vi "Convert_ERDs_Brass.vi"(0 "New Header?":bool, 7 "Array":T7[](array[typedef]) {"ERD Number" format="%.0x"}, 11 "Error In":errorcluster) -> (4 "All_ERD_Data_Bundled_Brass":T1, 15 "Error Out":errorcluster)   [LabVIEW 2016]
doc: "This VI parses the data from ERDs in correct format, units, etc. It handles all hex to dec conversions, hex to enum, and hex to boolean conversions.\n\nIf Raw Data from ERD is blank string, then it will output values from shift register."
uses:
  Common/LabVIEW GEA2 Toolkit/LabVIEW_GEA2_Toolkit.lvlibp/type defs/ERD Read Data Out.ctl
  type defs2/All_Bundled_Data_Brass.ctl
  Laundry Tool 1.0 Support/type defs/Version.ctl
  type defs2/ERD_Always_Show_Brass.ctl
  type defs2/CSV_File_String_Arrays.ctl
  type defs2/Fault Table Array.ctl
  Laundry Tool 1.0 Support/type defs/Fault_Table_Info.ctl
  Common/LabVIEW GEA2 Toolkit/LabVIEW_GEA2_Toolkit.lvlibp
panel:
  # "Software Version"
  # "UI - Critical Version"
  # "UI - Non-Critical"
  # "MC -  Version"
  # "Inverter Version"
  # "Model Setting"
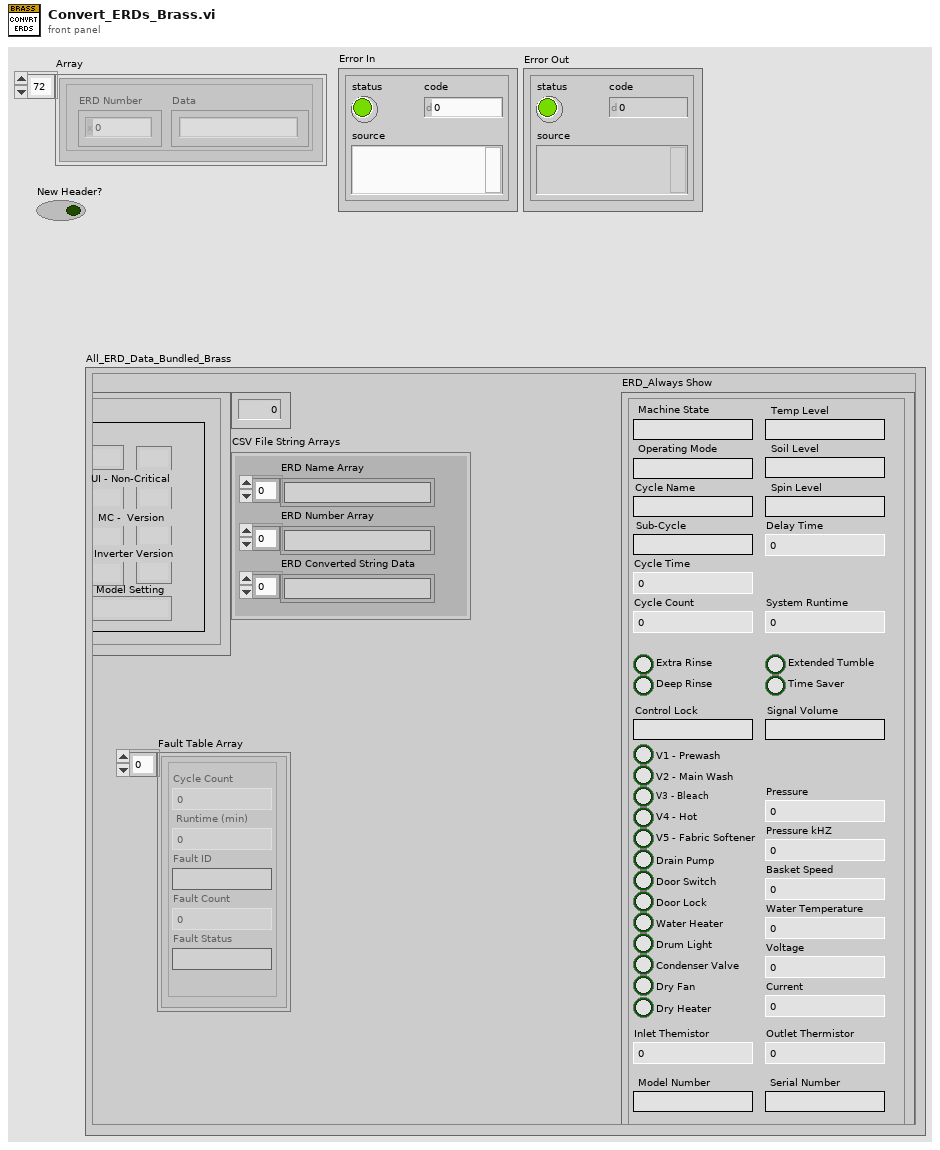
[diagram p1: front panel]
types:
  T1 = typedef "All_Bundled_Data_Brass.ctl" = cluster{"Version":T2, "ERD_Always Show":T3, "Personality Set":u8, "CSV File String Arrays":T4, "Fault Table Array ":T5}
  T2 = typedef "Version.ctl" = cluster{"UI - Critical Major":string, "UI - Critical Minor":string, "UI - Non-Critical Minor":string, "UI - Non-Critical Major":string, "MC Minor":string, "MC Major":string, "Model Setting":string, "Inverter Version  Minor":string, "Inverter Version Major":string}
  T3 = typedef "ERD_Always_Show_Brass.ctl" = cluster{"Machine State":string, "Cycle Count":u32, "Soil Level":string, "Spin Level":string, "Temp Level":string, "Delay Time":u16, "Sub-Cycle":string, "Cycle Name":string, "Model Number":string, "Serial Number":string, "System Runtime":u32, "Cycle Time":u16, "Operating Mode":string, "Deep Rinse":bool, "Extra Rinse":bool, "V1 - Prewash":bool, "V2 - Main Wash":bool, "V3 - Bleach":bool, "V4 - Hot":bool, "Drain Pump":bool, "Door Switch":bool, "Door Lock":bool, "Basket Speed":u16, "Water Temperature":dbl, "Voltage":dbl, "Pressure":dbl, "Water Heater":bool, "Control Lock":string, "Signal Volume":string, "Current":u16, "Pressure kHZ":dbl, "Drum Light":bool, "V5 - Fabric Softener":bool, "Inlet Themistor":dbl, "Outlet Thermistor":dbl, "Condenser Valve":bool, "Dry Fan":bool, "Dry Heater":bool, "Extended Tumble":bool, "Time Saver":bool}
  T4 = typedef "CSV_File_String_Arrays.ctl" = cluster{"ERD Number Array":string[], "ERD Name Array":string[], "ERD Converted String Data":string[]}
  T5 = typedef "Fault Table Array.ctl" = T6[]
  T6 = typedef "Fault_Table_Info.ctl" = cluster{"Cycle Count":u32, " Runtime (min) ":u32, "Fault Status":string, "Fault ID":string, "Fault Count":u16}
  T7 = typedef "LabVIEW_GEA2_Toolkit.lvlibp/ERD Read Data Out.ctl" = cluster{"ERD Number":u16, "Data":string}
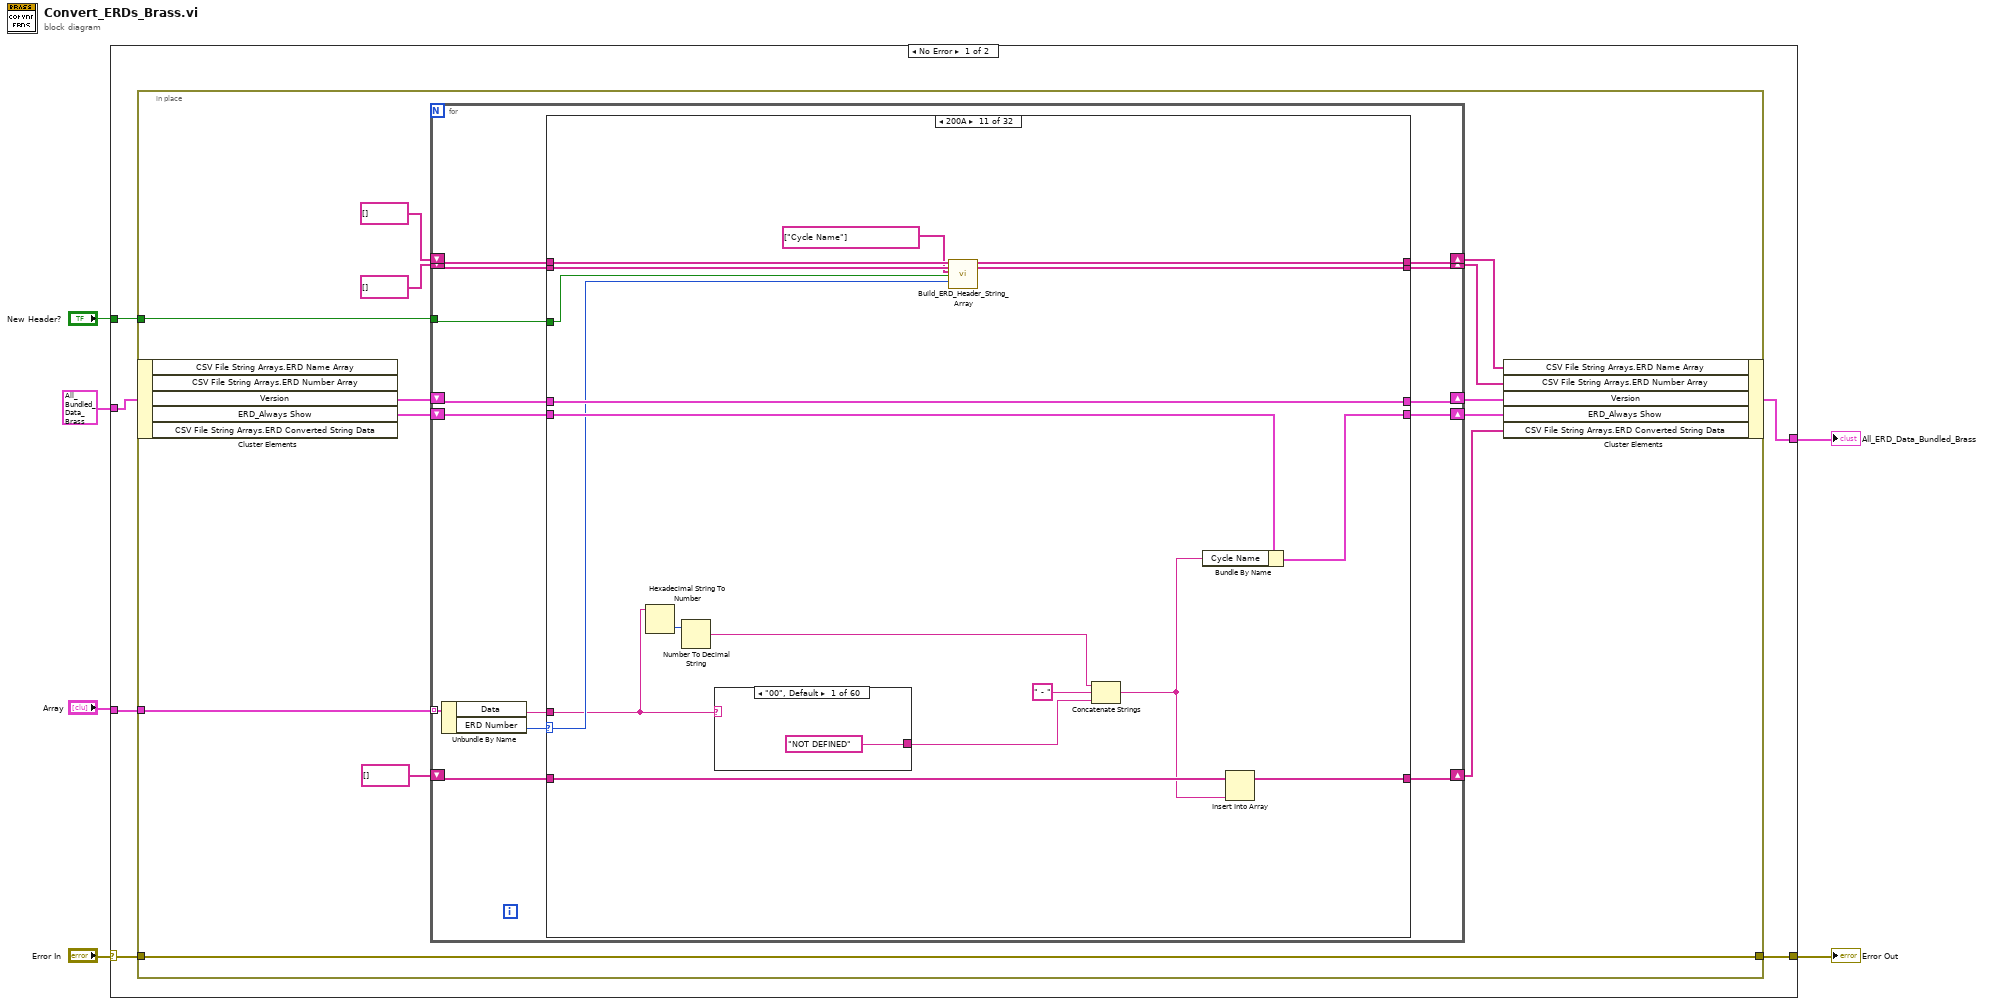
[diagram p0: block diagram]
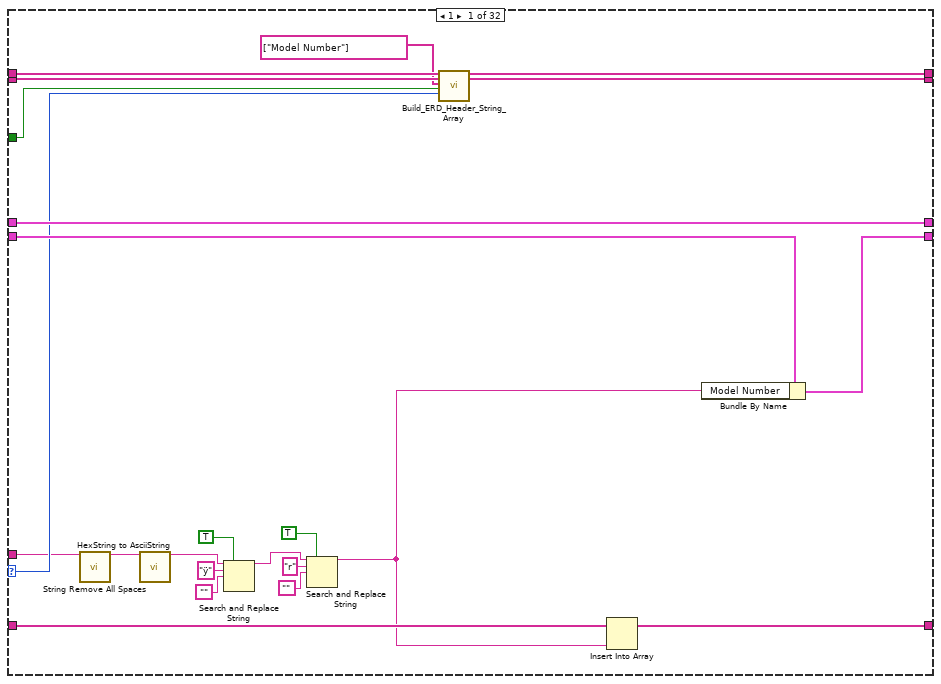
[diagram p2: hidden frame]
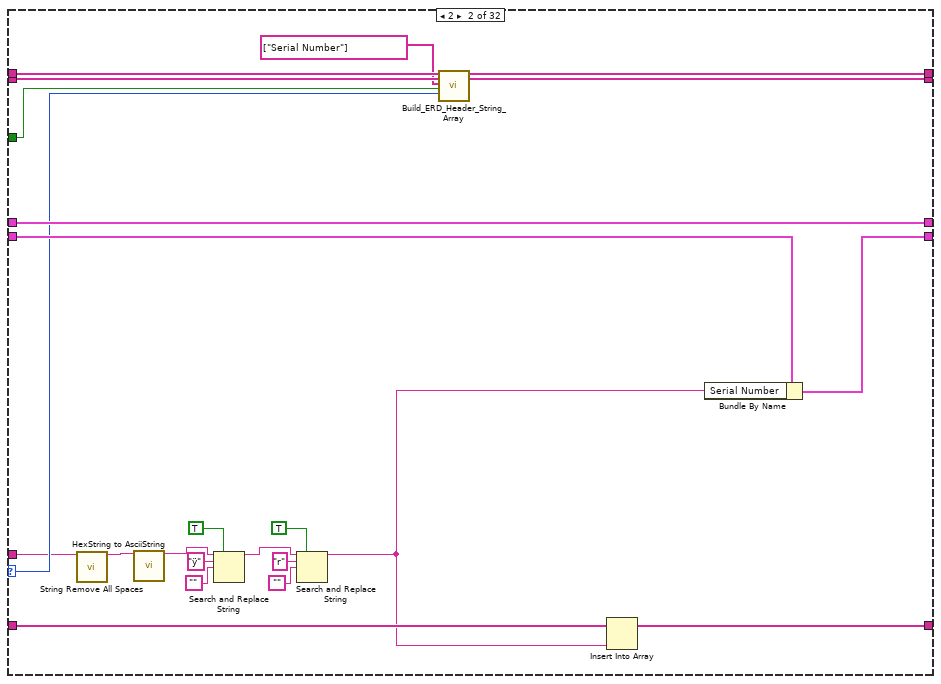
[diagram p3: hidden frame]
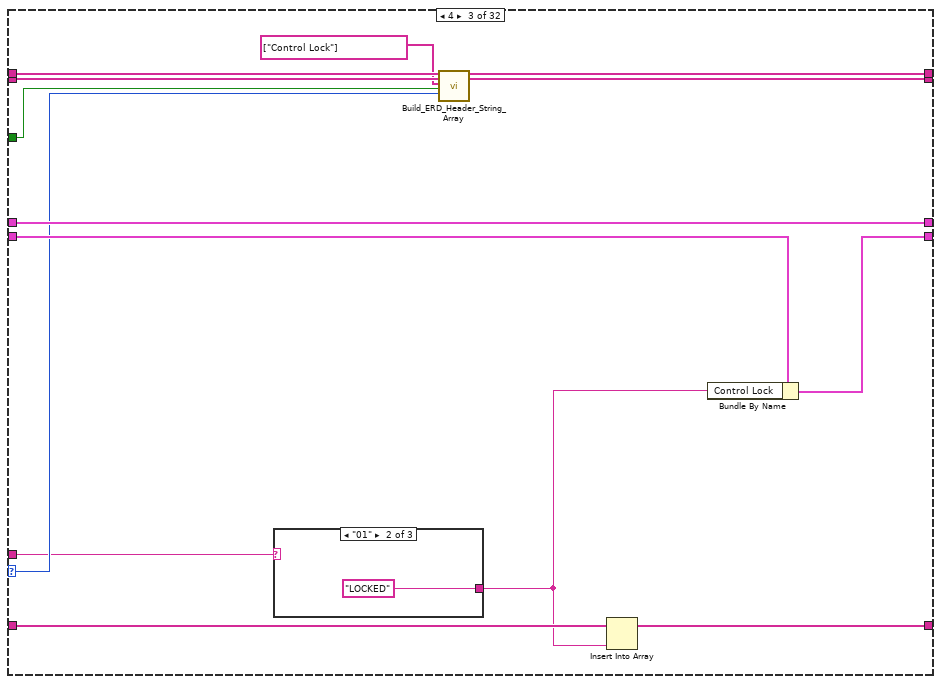
[diagram p4: hidden frame]
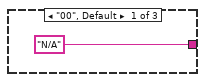
[diagram p5: hidden frame]
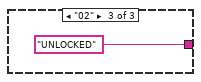
[diagram p6: hidden frame]
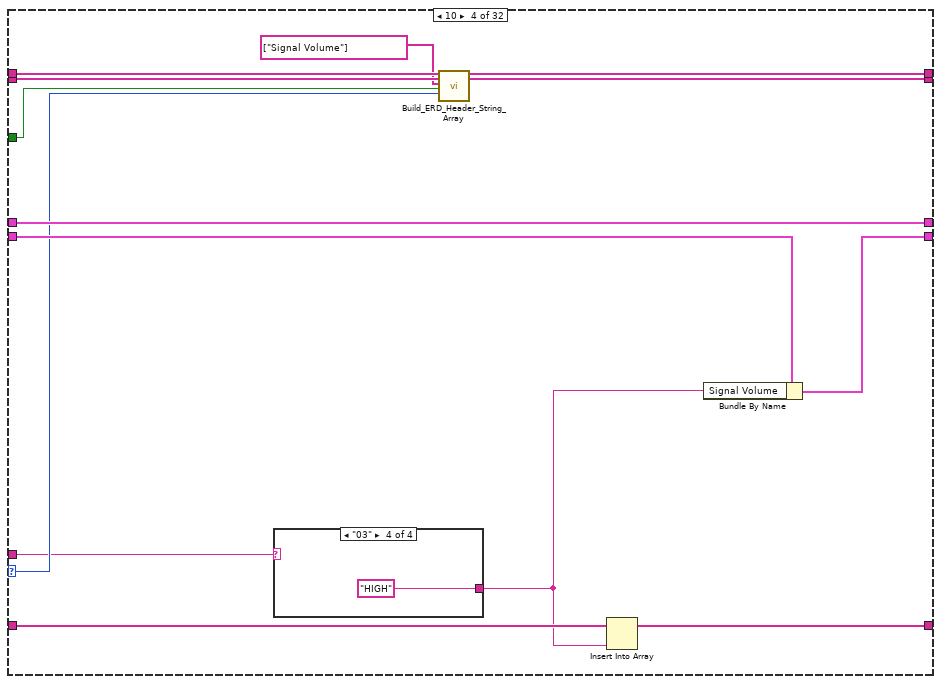
[diagram p7: hidden frame]
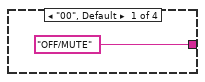
[diagram p8: hidden frame]
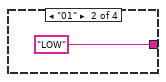
[diagram p9: hidden frame]
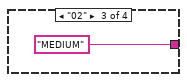
[diagram p10: hidden frame]
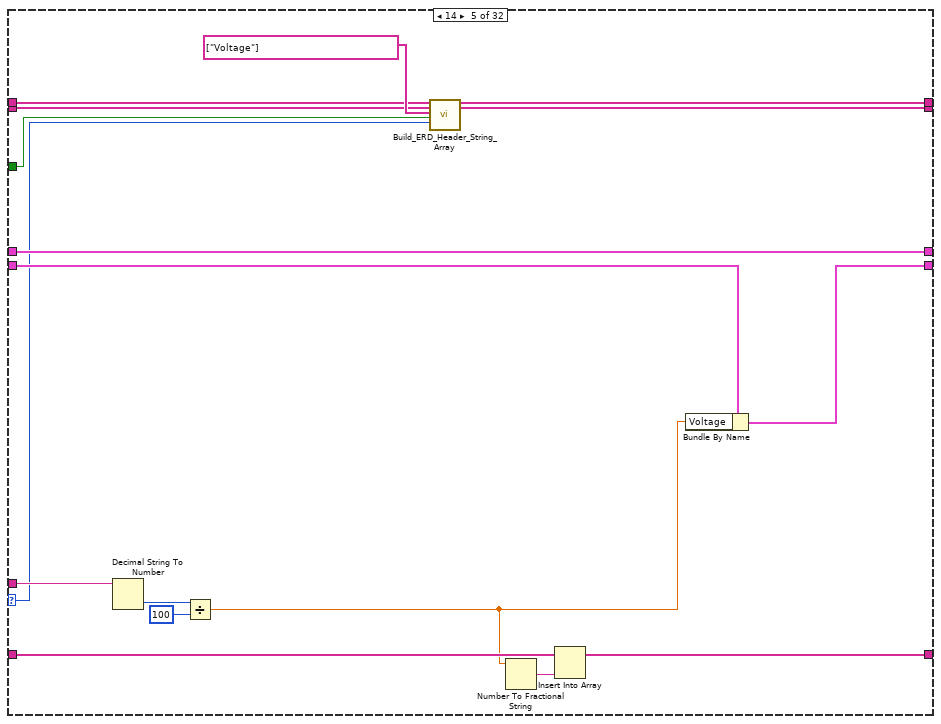
[diagram p11: hidden frame]
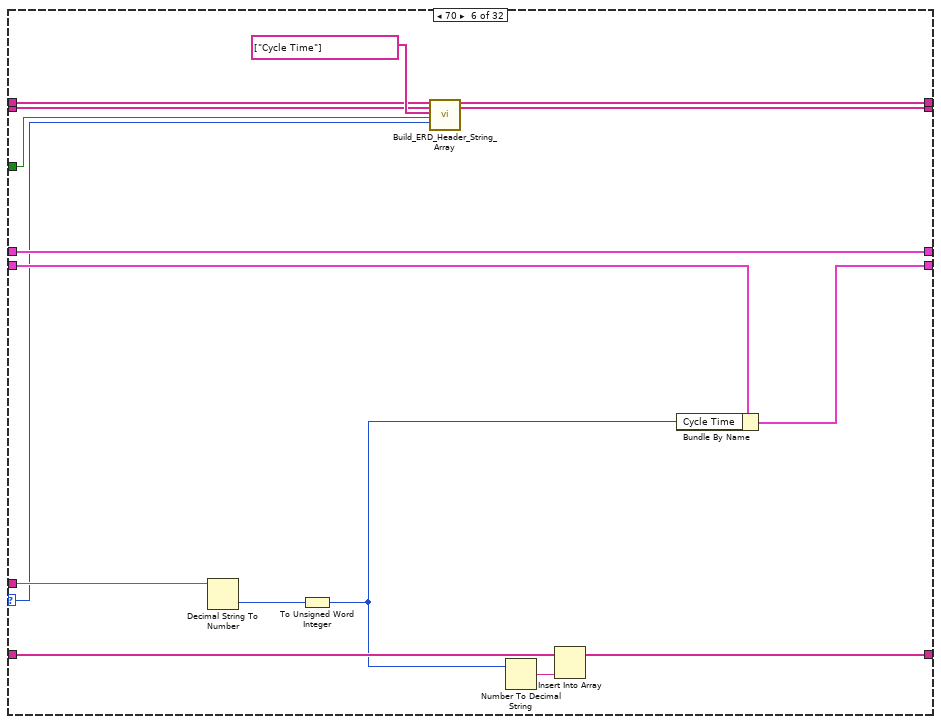
[diagram p12: hidden frame]
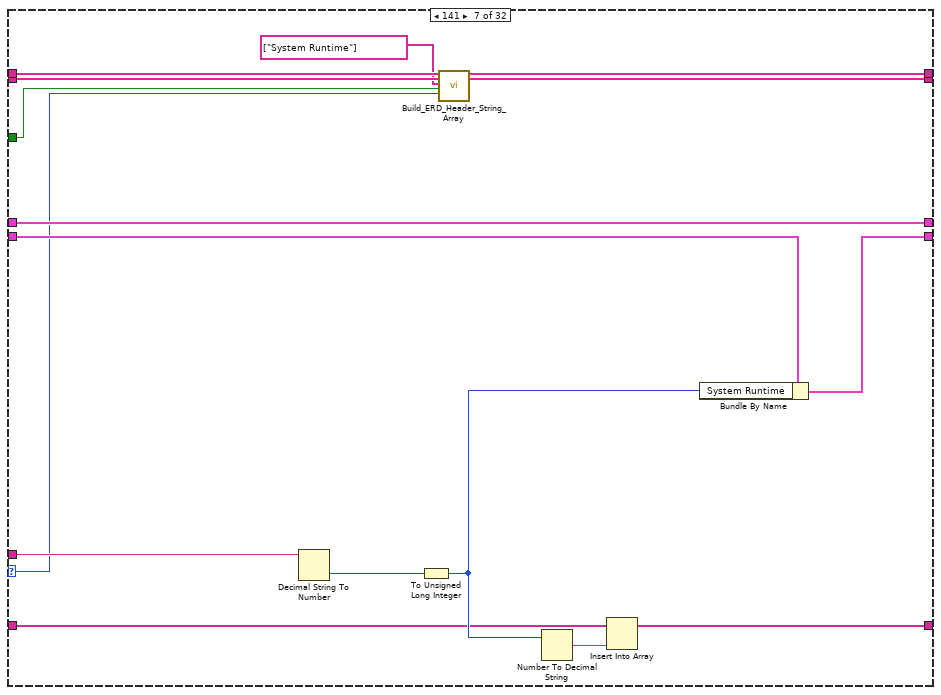
[diagram p13: hidden frame]
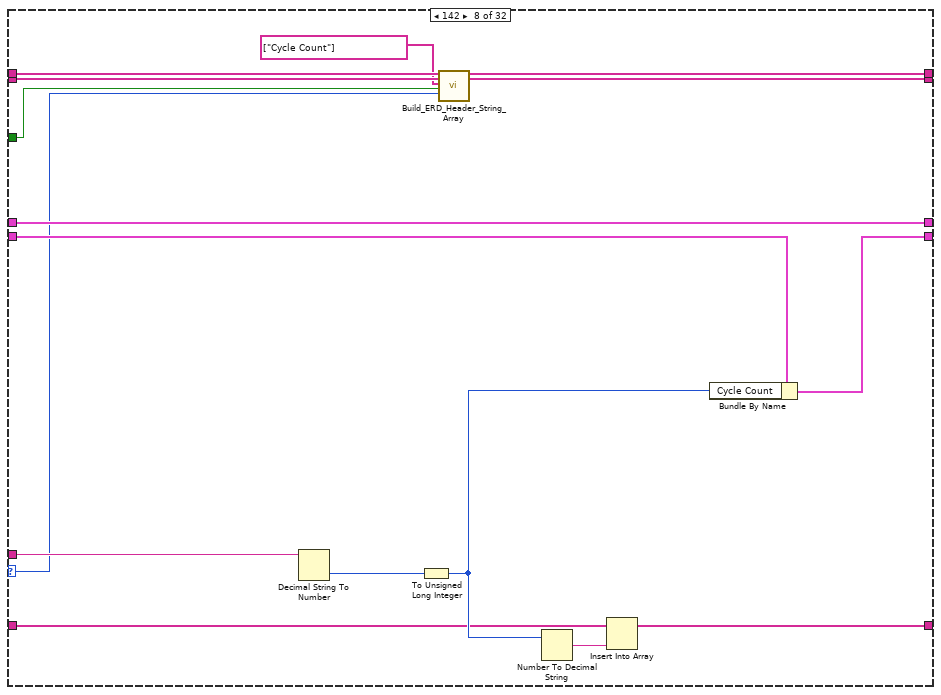
[diagram p14: hidden frame]
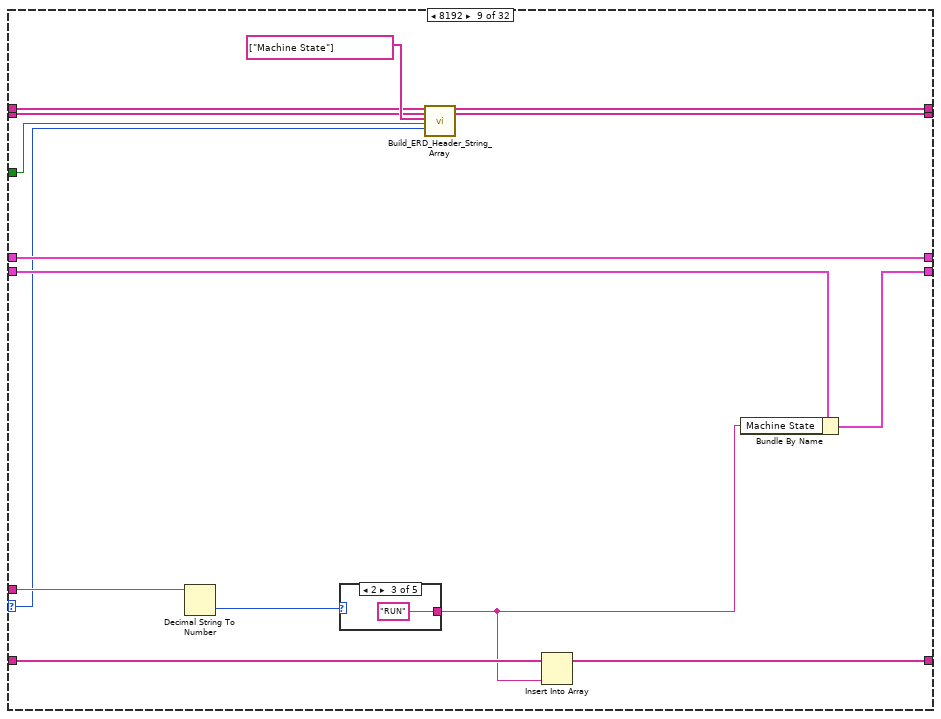
[diagram p15: hidden frame]
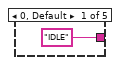
[diagram p16: hidden frame]
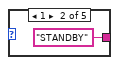
[diagram p17: hidden frame]
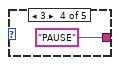
[diagram p18: hidden frame]
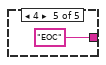
[diagram p19: hidden frame]
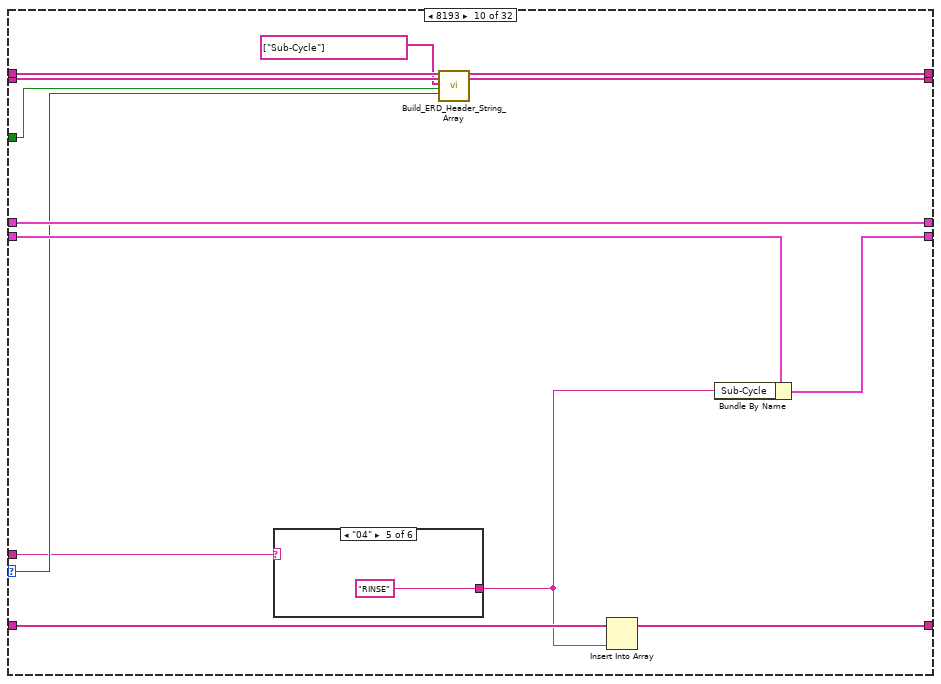
[diagram p20: hidden frame]
diagram:
  n1 = case shown="No Error" "Error In" {
    selector: "Error In" -> [w9 w798]
    tunnel: "Array" -> [w12 _]
    tunnel: [w10 w797] -> w4
    tunnel: T1 {"Version"={"UI - Critical Major"="", "UI - Critical Minor"="", "UI - Non-Critical Minor"="", "UI - Non-Critical Major"="", "MC Minor"="", "MC Major"="", "Model Setting"="", "Inverter Version  Minor"="", "Inverter Version Major"=""}, "ERD_Always Show"={"Machine State"="", "Cycle Count"=0, "Soil Level"="", "Spin Level"="", "Temp Level"="", "Delay Time"=0, "Sub-Cycle"="", "Cycle Name"="", "Model Number"="", "Serial Number"="", "System Runtime"=0, "Cycle Time"=0, "Operating Mode"="", "Deep Rinse"=FALSE, "Extra Rinse"=FALSE, "V1 - Prewash"=FALSE, "V2 - Main Wash"=FALSE, "V3 - Bleach"=FALSE, "V4 - Hot"=FALSE, "Drain Pump"=FALSE, "Door Switch"=FALSE, "Door Lock"=FALSE, "Basket Speed"=0, "Water Temperature"=0.0, "Voltage"=0.0, "Pressure"=0.0, "Water Heater"=FALSE, "Control Lock"="", "Signal Volume"="", "Current"=0, "Pressure kHZ"=0.0, "Drum Light"=FALSE, "V5 - Fabric Softener"=FALSE, "Inlet Themistor"=0.0, "Outlet Thermistor"=0.0, "Condenser Valve"=FALSE, "Dry Fan"=FALSE, "Dry Heater"=FALSE, "Extended Tumble"=FALSE, "Time Saver"=FALSE}, "Personality Set"=0, "CSV File String Arrays"={"ERD Number Array"=[], "ERD Name Array"=[], "ERD Converted String Data"=[]}, "Fault Table Array "=[]} ("ERD_Data_Bundled_Out") -> [w11 w796]
    tunnel: [w8 w796] -> w3
    tunnel: "New Header?" -> [w7 _]
    frame No Error {
      n2 = in-place {
        in-place-border: w12 -> [w25]
        in-place-border: [w22] -> w10
        in-place-border: w9 -> [w22]
        in-place-border: w7 -> [w18]
        n3 = in-place-cluster #1(w11) -> ("Version"=w23:T2, "ERD_Always Show"=w24:T3)  [unwired: 3 out]
        n4 = for {
          tunnel: w25 -> [w39] mode=indexing
          shift-right: [w37] -> w20
          shift-left: w24 -> [w36]
          shift-right: [w34] -> w21
          shift-left: w23 -> [w35]
          shift-right: [w31] -> w13
          shift-left: string[] [] ("ERD String Data") -> [w32]
          tunnel: w18 -> [w30]
          shift-right: [w26] -> w14
          shift-left: string[] [] ("ERD String Data") -> [w29]
          shift-right: [w27] -> w15
          shift-left: string[] [] ("ERD String Data") -> [w28]
          n5 = Unbundle By Name(w39) -> ("Data"=w38:string, "ERD Number"=w33:u16)
          n6 = case shown="200A" w33 {
            selector: w33 -> [w53 w76 w90 w107 w124 w138 w159 w175 w189 w210 w234 w308 w328 w349 w368 w382 w402 w425 w449 w477 w496 w513 w532 w551 w570 w593 w642 w685 w731 w760 w777 _]
            tunnel: w38 -> [w50 w73 w87 w104 w137 w152 w169 w185 w197 w207 w230 w305 w342 w346 w365 w393 w413 w436 w459 w491 w509 w526 w529 w548 w567 w592 w641 w698 w704 w773 w790 _]
            tunnel: [w61 w84 w98 w115 w135 w150 w167 w183 w200 w218 w242 w316 w340 w357 w376 w394 w414 w437 w460 w489 w507 w524 w540 w559 w578 w603 w652 w696 w742 w771 w788 w795] -> w37
            tunnel: w36 -> [w62 w85 w99 w116 w136 w151 w168 w184 w199 w219 w243 w317 w341 w358 w377 w395 w415 w438 w461 w490 w508 w525 w541 w560 w579 w604 w653 w697 w742 w772 w789 w795]
            tunnel: w35 -> [w60 w83 w97 w114 w134 w149 w166 w182 w196 w217 w241 w315 w339 w356 w375 w392 w412 w435 w458 w488 w506 w523 w539 w558 w577 w602 w651 w695 w744 w770 w787 w794]
            tunnel: [w60 w83 w97 w114 w134 w149 w166 w182 w196 w217 w241 w315 w339 w356 w375 w392 w412 w435 w458 w488 w506 w523 w539 w558 w577 w602 w651 w695 w743 w770 w787 w794] -> w34
            tunnel: w32 -> [w58 w81 w95 w112 w128 w142 w164 w180 w193 w215 w239 w313 w332 w354 w373 w386 w406 w429 w453 w481 w500 w517 w537 w556 w575 w597 w646 w689 w711 w764 w781 w792]
            tunnel: [w56 w79 w93 w110 w126 w140 w162 w178 w191 w213 w237 w311 w330 w352 w371 w384 w404 w427 w451 w479 w498 w515 w535 w554 w573 w595 w644 w687 w733 w762 w779 w792] -> w31
            tunnel: w30 -> [w54 w77 w91 w108 w125 w139 w160 w176 w190 w211 w235 w309 w329 w350 w369 w383 w403 w426 w450 w478 w497 w514 w533 w552 w571 w594 w643 w686 w732 w761 w778 _]
            tunnel: w29 -> [w59 w82 w96 w113 w129 w143 w165 w181 w194 w216 w240 w314 w333 w355 w374 w387 w407 w430 w454 w482 w501 w518 w538 w557 w576 w598 w647 w690 w735 w765 w782 w793]
            tunnel: w28 -> [w52 w75 w89 w106 w132 w147 w155 w171 w188 w209 w233 w307 w337 w348 w367 w391 w411 w434 w457 w486 w504 w521 w531 w550 w569 w601 w650 w693 w738 w768 w785 w791]
            tunnel: [w51 w74 w88 w105 w131 w146 w154 w170 w187 w208 w232 w306 w336 w347 w366 w390 w410 w433 w456 w485 w503 w520 w530 w549 w568 w600 w649 w692 w737 w767 w784 w791] -> w27
            tunnel: [w57 w80 w94 w111 w127 w141 w163 w179 w192 w214 w238 w312 w331 w353 w372 w385 w405 w428 w452 w480 w499 w516 w536 w555 w574 w596 w645 w688 w734 w763 w780 w793] -> w26
            frame 1 {
              n7 = call "String Remove All Spaces.vi"("Input String"=w50) -> ("Spaces Removed"=w49:string)  [unwired: 13 in, 1 out]
              n8 = call "HexString to AsciiString.vi"("Hex String"=w49) -> ("ASCII String"=w45:string)  [unwired: 13 in, 1 out]
              n9 = Search and Replace String(replace all?=TRUE ("replace all? (F)"), input string=w45, search string="ÿ", replace string="") -> (result string=w41:string)  [unwired: 4 in, 3 out]
              n10 = Search and Replace String(replace all?=TRUE ("replace all? (F)"), input string=w41, search string="r", replace string="") -> (result string=w44:string)  [unwired: 4 in, 3 out]
              n11 = call "Build_ERD_Header_String_Array.vi"("ERD Name Array In"=w59, "ERD Number Array In"=w58, "ERD Name List"=string[] ["Model Number"], "New Header?"=w54, "ERD Number"=w53) -> ("ERD Name Array Out"=w57:string[], "ERD Number Array Out"=w56:string[])  [unwired: 13 in]
              n12 = Insert Into Array(array=w52, new element=w44) -> (w51:string[])  [unwired: 1 in]
              n13 = Bundle By Name(cluster=w62, "Model Number"=w44) -> (w61:T3)
            }
            frame 2 {
              n14 = call "String Remove All Spaces.vi"("Input String"=w73) -> ("Spaces Removed"=w72:string)  [unwired: 13 in, 1 out]
              n15 = call "HexString to AsciiString.vi"("Hex String"=w72) -> ("ASCII String"=w69:string)  [unwired: 13 in, 1 out]
              n16 = Search and Replace String(replace all?=TRUE ("replace all? (F)"), input string=w69, search string="ÿ", replace string="") -> (result string=w64:string)  [unwired: 4 in, 3 out]
              n17 = Search and Replace String(replace all?=TRUE ("replace all? (F)"), input string=w64, search string="r", replace string="") -> (result string=w63:string)  [unwired: 4 in, 3 out]
              n18 = call "Build_ERD_Header_String_Array.vi"("ERD Name Array In"=w82, "ERD Number Array In"=w81, "ERD Name List"=string[] ["Serial Number"], "New Header?"=w77, "ERD Number"=w76) -> ("ERD Name Array Out"=w80:string[], "ERD Number Array Out"=w79:string[])  [unwired: 13 in]
              n19 = Insert Into Array(array=w75, new element=w63) -> (w74:string[])  [unwired: 1 in]
              n20 = Bundle By Name(cluster=w85, "Serial Number"=w63) -> (w84:T3)
            }
            frame 4 {
              n21 = case shown="\"01\"" w87 {
                tunnel: ["N/A" "LOCKED" "UNLOCKED"] -> w86
                frame "00", Default {
                }
                frame "01" {
                }
                frame "02" {
                }
              }
              n22 = call "Build_ERD_Header_String_Array.vi"("ERD Name Array In"=w96, "ERD Number Array In"=w95, "ERD Name List"=string[] ["Control Lock"], "New Header?"=w91, "ERD Number"=w90) -> ("ERD Name Array Out"=w94:string[], "ERD Number Array Out"=w93:string[])  [unwired: 13 in]
              n23 = Insert Into Array(array=w89, new element=w86) -> (w88:string[])  [unwired: 1 in]
              n24 = Bundle By Name(cluster=w99, "Control Lock"=w86) -> (w98:T3)
            }
            frame 10 {
              n25 = case shown="\"03\"" w104 {
                tunnel: ["OFF/MUTE" "LOW" "MEDIUM" "HIGH"] -> w103
                frame "00", Default {
                }
                frame "01" {
                }
                frame "02" {
                }
                frame "03" {
                }
              }
              n26 = call "Build_ERD_Header_String_Array.vi"("ERD Name Array In"=w113, "ERD Number Array In"=w112, "ERD Name List"=string[] ["Signal Volume"], "New Header?"=w108, "ERD Number"=w107) -> ("ERD Name Array Out"=w111:string[], "ERD Number Array Out"=w110:string[])  [unwired: 13 in]
              n27 = Insert Into Array(array=w106, new element=w103) -> (w105:string[])  [unwired: 1 in]
              n28 = Bundle By Name(cluster=w116, "Signal Volume"=w103) -> (w115:T3)
            }
            frame 14 {
              n29 = Decimal String To Number(string=w137) -> (number=w123:i32)  [unwired: 2 in, 1 out]
              n30 = Divide(x=w123, y=100) -> (x/y=w121:dbl)
              n31 = call "Build_ERD_Header_String_Array.vi"("ERD Name Array In"=w129, "ERD Number Array In"=w128, "ERD Name List"=string[] ["Voltage"], "New Header?"=w125, "ERD Number"=w124) -> ("ERD Name Array Out"=w127:string[], "ERD Number Array Out"=w126:string[])  [unwired: 13 in]
              n32 = Number To Fractional String(number=w121) -> (F-format string=w133:string)  [unwired: 3 in]
              n33 = Insert Into Array(array=w132, new element=w133) -> (w131:string[])  [unwired: 1 in]
              n34 = Bundle By Name(cluster=w136, "Voltage"=w121) -> (w135:T3)
            }
            frame 70 {
              n35 = Decimal String To Number(string=w152) -> (number=w153:i32)  [unwired: 2 in, 1 out]
              n36 = To Unsigned Word Integer(number=w153) -> (unsigned 16bit integer=w145:u16)
              n37 = call "Build_ERD_Header_String_Array.vi"("ERD Name Array In"=w143, "ERD Number Array In"=w142, "ERD Name List"=string[] ["Cycle Time"], "New Header?"=w139, "ERD Number"=w138) -> ("ERD Name Array Out"=w141:string[], "ERD Number Array Out"=w140:string[])  [unwired: 13 in]
              n38 = Number To Decimal String(number=w145) -> (decimal integer string=w148:string)  [unwired: 1 in]
              n39 = Insert Into Array(array=w147, new element=w148) -> (w146:string[])  [unwired: 1 in]
              n40 = Bundle By Name(cluster=w151, "Cycle Time"=w145) -> (w150:T3)
            }
            frame 141 {
              n41 = Decimal String To Number(string=w169) -> (number=w157:i32)  [unwired: 2 in, 1 out]
              n42 = To Unsigned Long Integer(number=w157) -> (unsigned 32bit integer=w156:u32)
              n43 = call "Build_ERD_Header_String_Array.vi"("ERD Name Array In"=w165, "ERD Number Array In"=w164, "ERD Name List"=string[] ["System Runtime"], "New Header?"=w160, "ERD Number"=w159) -> ("ERD Name Array Out"=w163:string[], "ERD Number Array Out"=w162:string[])  [unwired: 13 in]
              n44 = Number To Decimal String(number=w156) -> (decimal integer string=w158:string)  [unwired: 1 in]
              n45 = Insert Into Array(array=w155, new element=w158) -> (w154:string[])  [unwired: 1 in]
              n46 = Bundle By Name(cluster=w168, "System Runtime"=w156) -> (w167:T3)
            }
            frame 142 {
              n47 = Decimal String To Number(string=w185) -> (number=w173:i32)  [unwired: 2 in, 1 out]
              n48 = To Unsigned Long Integer(number=w173) -> (unsigned 32bit integer=w172:u32)
              n49 = call "Build_ERD_Header_String_Array.vi"("ERD Name Array In"=w181, "ERD Number Array In"=w180, "ERD Name List"=string[] ["Cycle Count"], "New Header?"=w176, "ERD Number"=w175) -> ("ERD Name Array Out"=w179:string[], "ERD Number Array Out"=w178:string[])  [unwired: 13 in]
              n50 = Number To Decimal String(number=w172) -> (decimal integer string=w174:string)  [unwired: 1 in]
              n51 = Insert Into Array(array=w171, new element=w174) -> (w170:string[])  [unwired: 1 in]
              n52 = Bundle By Name(cluster=w184, "Cycle Count"=w172) -> (w183:T3)
            }
            frame 8192 {
              n53 = Decimal String To Number(string=w197) -> (number=w198:i32)  [unwired: 2 in, 1 out]
              n54 = case shown="2" w198 {
                tunnel: ["IDLE" "STANDBY" "RUN" "PAUSE" "EOC"] -> w186
                frame 0, Default {
                }
                frame 1 {
                }
                frame 2 {
                }
                frame 3 {
                }
                frame 4 {
                }
              }
              n55 = call "Build_ERD_Header_String_Array.vi"("ERD Name Array In"=w194, "ERD Number Array In"=w193, "ERD Name List"=string[] ["Machine State"], "New Header?"=w190, "ERD Number"=w189) -> ("ERD Name Array Out"=w192:string[], "ERD Number Array Out"=w191:string[])  [unwired: 13 in]
              n56 = Insert Into Array(array=w188, new element=w186) -> (w187:string[])  [unwired: 1 in]
              n57 = Bundle By Name(cluster=w199, "Machine State"=w186) -> (w200:T3)
            }
            frame 8193 {
              n58 = case shown="\"04\"" w207 {
                tunnel: ["N/A" "FILL" "SOAK" "WASH" "RINSE" "SPIN"] -> w206
                frame "00", Default {
                }
                frame "01" {
                }
                frame "02" {
                }
                frame "03" {
                }
                frame "04" {
                }
                frame "05" {
                }
              }
              n59 = call "Build_ERD_Header_String_Array.vi"("ERD Name Array In"=w216, "ERD Number Array In"=w215, "ERD Name List"=string[] ["Sub-Cycle"], "New Header?"=w211, "ERD Number"=w210) -> ("ERD Name Array Out"=w214:string[], "ERD Number Array Out"=w213:string[])  [unwired: 13 in]
              n60 = Insert Into Array(array=w209, new element=w206) -> (w208:string[])  [unwired: 1 in]
              n61 = Bundle By Name(cluster=w219, "Sub-Cycle"=w206) -> (w218:T3)
            }
            frame 8202 {
              n62 = Hexadecimal String To Number(string=w230) -> (number=w231:u32)  [unwired: 2 in, 1 out]
              n63 = Number To Decimal String(number=w231) -> (decimal integer string=w227:string)  [unwired: 1 in]
              n64 = case shown="\"00\", Default" w230 {
                tunnel: ["NOT DEFINED" "BASKET CLEAN" "DRAIN & SPN" "QUICK RINSE" "BULKY ITEMS" "SANITIZE" "TOWELS & SHEETS" "STEAM REFRESH" "NORMAL/MIXED" "WHITES" "DARK COLORS" "JEANS" "HAND WASH" "DELICATES" "SPEED WASH" "HEAVY DUTY" "ALLERGEN" "POWER CLEAN" "RINSE & SPIN" "SINGLE ITEM" "COLORS" "COLD WASH" "WATER STATION" "TUB CLEAN" "CASUALS W/ STEAM" "STAIN WASH W/ STEAM" "DEEP CLEAN" "BULKY BEDDING" "NORMAL" "QUICK WASH" "SANITIZE W/ OXI" "SELF CLEAN" "TOWELS" "SOAK" "WOOL" "ULTRA FRESH VENT" "SANITIZE & ALLERGEN" "SPIN ONLY" "COTTONS" "EASY CARE" "ACTIVE WEAR" "TIMED DRY" "DEWRINKLE" "AIR FLUFF" "STEAM REFRESH" "STEAM DEWRINKLE" "SPEED DRY" "MIXED" "QUICK DRY" "CASUALS" "WARM UP" "ENERGY SAVER" "ANTIBACTERIAL" "RACK DRY" "BABY CARE" "AUTO DRY" "AUTO EXTRA DRY" "PERM PRESS" "WASHER LINK" "AUTO DAMP DRY"] -> w229
                frame "00", Default {
                }
                frame "01" {
                }
                frame "02" {
                }
                frame "03" {
                }
                frame "04" {
                }
                frame "05" {
                }
                frame "06" {
                }
                frame "07" {
                }
                frame "08" {
                }
                frame "09" {
                }
                frame "0A" {
                }
                frame "0B" {
                }
                frame "0C" {
                }
                frame "0D" {
                }
                frame "0E" {
                }
                frame "0F" {
                }
                frame "10" {
                }
                frame "11" {
                }
                frame "12" {
                }
                frame "13" {
                }
                frame "14" {
                }
                frame "15" {
                }
                frame "16" {
                }
                frame "17" {
                }
                frame "18" {
                }
                frame "19" {
                }
                frame "1A" {
                }
                frame "1B" {
                }
                frame "1C" {
                }
                frame "1D" {
                }
                frame "1E" {
                }
                frame "1F" {
                }
                frame "20" {
                }
                frame "21" {
                }
                frame "22" {
                }
                frame "23" {
                }
                frame "24" {
                }
                frame "25" {
                }
                frame "80" {
                }
                frame "81" {
                }
                frame "82" {
                }
                frame "83" {
                }
                frame "84" {
                }
                frame "85" {
                }
                frame "86" {
                }
                frame "87" {
                }
                frame "88" {
                }
                frame "89" {
                }
                frame "8A" {
                }
                frame "8B" {
                }
                frame "8C" {
                }
                frame "8D" {
                }
                frame "8E" {
                }
                frame "8F" {
                }
                frame "90" {
                }
                frame "91" {
                }
                frame "92" {
                }
                frame "93" {
                }
                frame "94" {
                }
                frame "95" {
                }
              }
              n65 = call "Build_ERD_Header_String_Array.vi"("ERD Name Array In"=w240, "ERD Number Array In"=w239, "ERD Name List"=string[] ["Cycle Name"], "New Header?"=w235, "ERD Number"=w234) -> ("ERD Name Array Out"=w238:string[], "ERD Number Array Out"=w237:string[])  [unwired: 13 in]
              n66 = Concatenate Strings(w227, " - " ("string"), w229) -> (w228:string)
              n67 = Bundle By Name(cluster=w243, "Cycle Name"=w228) -> (w242:T3)
              n68 = Insert Into Array(array=w233, new element=w228) -> (w232:string[])  [unwired: 1 in]
            }
            frame 8206 {
              n69 = case shown="\"08\"" w305 {
                tunnel: ["CONSUMER MODE" "SERVICE MODE" "FACTORY/EOL MODE" "CONTINUOUS CYCLE MODE" "RAPID RELAY MODE" "FCT MODE" "MODEL PLUG" "DEMO MODE" "CONSUMER ERROR MODE" "FLOOR TYPE SELECTION MODE"] -> w304
                frame "00", Default {
                }
                frame "01" {
                }
                frame "02" {
                }
                frame "03" {
                }
                frame "04" {
                }
                frame "05" {
                }
                frame "06" {
                }
                frame "07" {
                }
                frame "08" {
                }
                frame "09" {
                }
              }
              n70 = call "Build_ERD_Header_String_Array.vi"("ERD Name Array In"=w314, "ERD Number Array In"=w313, "ERD Name List"=string[] ["Operating Mode"], "New Header?"=w309, "ERD Number"=w308) -> ("ERD Name Array Out"=w312:string[], "ERD Number Array Out"=w311:string[])  [unwired: 13 in]
              n71 = Insert Into Array(array=w307, new element=w304) -> (w306:string[])  [unwired: 1 in]
              n72 = Bundle By Name(cluster=w317, "Operating Mode"=w304) -> (w316:T3)
            }
            frame 8208 {
              n73 = Decimal String To Number(string=w342) -> (number=w343:i32)  [unwired: 2 in, 1 out]
              n74 = To Unsigned Word Integer(number=w343) -> (unsigned 16bit integer=w335:u16)
              n75 = call "Build_ERD_Header_String_Array.vi"("ERD Name Array In"=w333, "ERD Number Array In"=w332, "ERD Name List"=string[] ["Delay Time"], "New Header?"=w329, "ERD Number"=w328) -> ("ERD Name Array Out"=w331:string[], "ERD Number Array Out"=w330:string[])  [unwired: 13 in]
              n76 = Number To Decimal String(number=w335) -> (decimal integer string=w338:string)  [unwired: 1 in]
              n77 = Insert Into Array(array=w337, new element=w338) -> (w336:string[])  [unwired: 1 in]
              n78 = Bundle By Name(cluster=w341, "Delay Time"=w335) -> (w340:T3)
            }
            frame 8210 {
              n79 = case shown="\"01\"" w346 {
                tunnel: ["OPEN" "CLOSED"] -> w345
                tunnel: [FALSE TRUE] -> w344
                frame "00", Default {
                }
                frame "01" {
                }
              }
              n80 = call "Build_ERD_Header_String_Array.vi"("ERD Name Array In"=w355, "ERD Number Array In"=w354, "ERD Name List"=string[] ["Door Switch"], "New Header?"=w350, "ERD Number"=w349) -> ("ERD Name Array Out"=w353:string[], "ERD Number Array Out"=w352:string[])  [unwired: 13 in]
              n81 = Insert Into Array(array=w348, new element=w345) -> (w347:string[])  [unwired: 1 in]
              n82 = Bundle By Name(cluster=w358, "Door Switch"=w344) -> (w357:T3)
            }
            frame 8211 {
              n83 = case shown="\"00\", Default" w365 {
                tunnel: ["UNLOCKED" "LOCKED"] -> w364
                tunnel: [FALSE TRUE] -> w363
                frame "00", Default {
                }
                frame "01" {
                }
              }
              n84 = call "Build_ERD_Header_String_Array.vi"("ERD Name Array In"=w374, "ERD Number Array In"=w373, "ERD Name List"=string[] ["Door Lock"], "New Header?"=w369, "ERD Number"=w368) -> ("ERD Name Array Out"=w372:string[], "ERD Number Array Out"=w371:string[])  [unwired: 13 in]
              n85 = Insert Into Array(array=w367, new element=w364) -> (w366:string[])  [unwired: 1 in]
              n86 = Bundle By Name(cluster=w377, "Door Lock"=w363) -> (w376:T3)
            }
            frame 8213 {
              n87 = case shown="\"00\"" w393 {
                selector: w393 -> [w396 _ _ _ _ _]
                tunnel: [w396 "EXTRA LIGHT" "LIGHT" "NORMAL" "HEAVY" "EXTRA HEAVY"] -> w389
                frame Default {
                }
                frame "00" {
                }
                frame "01" {
                }
                frame "02" {
                }
                frame "03" {
                }
                frame "04" {
                }
              }
              n88 = call "Build_ERD_Header_String_Array.vi"("ERD Name Array In"=w387, "ERD Number Array In"=w386, "ERD Name List"=string[] ["Soil Level"], "New Header?"=w383, "ERD Number"=w382) -> ("ERD Name Array Out"=w385:string[], "ERD Number Array Out"=w384:string[])  [unwired: 13 in]
              n89 = Insert Into Array(array=w391, new element=w389) -> (w390:string[])  [unwired: 1 in]
              n90 = Bundle By Name(cluster=w395, "Soil Level"=w389) -> (w394:T3)
            }
            frame 8214 {
              n91 = case shown="\"19\"" w413 {
                selector: w413 -> [w416 _ _ _ _ _ _ _ _]
                tunnel: [w416 "DISABLED" "TAP COLD" "COLD" "COOL" "COLORS" "WARM" "HOT" "EXTRA HOT"] -> w409
                frame Default {
                }
                frame "06" {
                }
                frame "16" {
                }
                frame "17" {
                }
                frame "18" {
                }
                frame "19" {
                }
                frame "20" {
                }
                frame "21" {
                }
                frame "22" {
                }
              }
              n92 = call "Build_ERD_Header_String_Array.vi"("ERD Name Array In"=w407, "ERD Number Array In"=w406, "ERD Name List"=string[] ["Temp Level"], "New Header?"=w403, "ERD Number"=w402) -> ("ERD Name Array Out"=w405:string[], "ERD Number Array Out"=w404:string[])  [unwired: 13 in]
              n93 = Insert Into Array(array=w411, new element=w409) -> (w410:string[])  [unwired: 1 in]
              n94 = Bundle By Name(cluster=w415, "Temp Level"=w409) -> (w414:T3)
            }
            frame 8215 {
              n95 = case shown="\"5\"" w436 {
                selector: w436 -> [w439 _ _ _ _ _ _]
                tunnel: [w439 "NO SPIN" "LOW" "MEDIUM" "HIGH" "EXTRA HIGH" "DISABLED"] -> w432
                frame Default {
                }
                frame "0" {
                }
                frame "1" {
                }
                frame "2" {
                }
                frame "3" {
                }
                frame "4" {
                }
                frame "5" {
                }
              }
              n96 = call "Build_ERD_Header_String_Array.vi"("ERD Name Array In"=w430, "ERD Number Array In"=w429, "ERD Name List"=string[] ["Spin Level"], "New Header?"=w426, "ERD Number"=w425) -> ("ERD Name Array Out"=w428:string[], "ERD Number Array Out"=w427:string[])  [unwired: 13 in]
              n97 = Insert Into Array(array=w434, new element=w432) -> (w433:string[])  [unwired: 1 in]
              n98 = Bundle By Name(cluster=w438, "Spin Level"=w432) -> (w437:T3)
            }
            frame 8216 {
              n99 = case shown="\"0\"" w459 {
                selector: w459 -> [w462 _ _ _ _]
                tunnel: [w462 "0 - DEEP RINSE OFF - EXTRA RINSE OFF" "1 - DEEP RINSE ON - EXTRA RINSE OFF" "2 - DEEP RINSE OFF - EXTRA RINSE ON" "3 - DEEP RINSE ON - EXTRA RINSE ON"] -> w448
                tunnel: [FALSE FALSE TRUE FALSE TRUE] -> w447
                tunnel: [FALSE FALSE FALSE TRUE TRUE] -> w446
                frame Default {
                }
                frame "0" {
                }
                frame "1" {
                }
                frame "2" {
                }
                frame "3" {
                }
              }
              n100 = call "Build_ERD_Header_String_Array.vi"("ERD Name Array In"=w454, "ERD Number Array In"=w453, "ERD Name List"=string[] ["Rinse Options"], "New Header?"=w450, "ERD Number"=w449) -> ("ERD Name Array Out"=w452:string[], "ERD Number Array Out"=w451:string[])  [unwired: 13 in]
              n101 = Insert Into Array(array=w457, new element=w448) -> (w456:string[])  [unwired: 1 in]
              n102 = Bundle By Name(cluster=w461, "Deep Rinse"=w447, "Extra Rinse"=w446) -> (w460:T3)
            }
            frame 8236 {
              n103 = Decimal String To Number(string=w491) -> (number=w492:i32)  [unwired: 2 in, 1 out]
              n104 = To Unsigned Word Integer(number=w492) -> (unsigned 16bit integer=w484:u16)
              n105 = call "Build_ERD_Header_String_Array.vi"("ERD Name Array In"=w482, "ERD Number Array In"=w481, "ERD Name List"=string[] ["Basket Speed"], "New Header?"=w478, "ERD Number"=w477) -> ("ERD Name Array Out"=w480:string[], "ERD Number Array Out"=w479:string[])  [unwired: 13 in]
              n106 = Number To Decimal String(number=w484) -> (decimal integer string=w487:string)  [unwired: 1 in]
              n107 = Insert Into Array(array=w486, new element=w487) -> (w485:string[])  [unwired: 1 in]
              n108 = Bundle By Name(cluster=w490, "Basket Speed"=w484) -> (w489:T3)
            }
            frame 8258 {
              n109 = Decimal String To Number(string=w509) -> (number=w495:i32)  [unwired: 2 in, 1 out]
              n110 = Divide(x=w495, y=1000) -> (x/y=w493:dbl)
              n111 = call "Build_ERD_Header_String_Array.vi"("ERD Name Array In"=w501, "ERD Number Array In"=w500, "ERD Name List"=string[] ["Pressure"], "New Header?"=w497, "ERD Number"=w496) -> ("ERD Name Array Out"=w499:string[], "ERD Number Array Out"=w498:string[])  [unwired: 13 in]
              n112 = Number To Fractional String(number=w493) -> (F-format string=w505:string)  [unwired: 3 in]
              n113 = Insert Into Array(array=w504, new element=w505) -> (w503:string[])  [unwired: 1 in]
              n114 = Bundle By Name(cluster=w508, "Pressure"=w493) -> (w507:T3)
            }
            frame 8259 {
              n115 = Decimal String To Number(string=w526) -> (number=w512:i32)  [unwired: 2 in, 1 out]
              n116 = Divide(x=w512, y=10) -> (x/y=w510:dbl)
              n117 = call "Build_ERD_Header_String_Array.vi"("ERD Name Array In"=w518, "ERD Number Array In"=w517, "ERD Name List"=string[] ["Water Temperature"], "New Header?"=w514, "ERD Number"=w513) -> ("ERD Name Array Out"=w516:string[], "ERD Number Array Out"=w515:string[])  [unwired: 13 in]
              n118 = Number To Fractional String(number=w510) -> (F-format string=w522:string)  [unwired: 3 in]
              n119 = Insert Into Array(array=w521, new element=w522) -> (w520:string[])  [unwired: 1 in]
              n120 = Bundle By Name(cluster=w525, "Water Temperature"=w510) -> (w524:T3)
            }
            frame 8275 {
              n121 = case shown="\"00\", Default" w529 {
                tunnel: ["OFF" "ON"] -> w528
                tunnel: [FALSE TRUE] -> w527
                frame "00", Default {
                }
                frame "01" {
                }
              }
              n122 = call "Build_ERD_Header_String_Array.vi"("ERD Name Array In"=w538, "ERD Number Array In"=w537, "ERD Name List"=string[] ["Extended Tumble"], "New Header?"=w533, "ERD Number"=w532) -> ("ERD Name Array Out"=w536:string[], "ERD Number Array Out"=w535:string[])  [unwired: 13 in]
              n123 = Insert Into Array(array=w531, new element=w528) -> (w530:string[])  [unwired: 1 in]
              n124 = Bundle By Name(cluster=w541, "Extended Tumble"=w527) -> (w540:T3)
            }
            frame 8277 {
              n125 = case shown="\"00\", Default" w548 {
                tunnel: ["OFF" "ON"] -> w547
                tunnel: [FALSE TRUE] -> w546
                frame "00", Default {
                }
                frame "01" {
                }
              }
              n126 = call "Build_ERD_Header_String_Array.vi"("ERD Name Array In"=w557, "ERD Number Array In"=w556, "ERD Name List"=string[] ["Tme Saver"], "New Header?"=w552, "ERD Number"=w551) -> ("ERD Name Array Out"=w555:string[], "ERD Number Array Out"=w554:string[])  [unwired: 13 in]
              n127 = Insert Into Array(array=w550, new element=w547) -> (w549:string[])  [unwired: 1 in]
              n128 = Bundle By Name(cluster=w560, "Time Saver"=w546) -> (w559:T3)
            }
            frame 61452 {
              n129 = case shown="\"00\", Default" w567 {
                tunnel: ["OFF" "ON"] -> w566
                tunnel: [FALSE TRUE] -> w565
                frame "00", Default {
                }
                frame "01" {
                }
              }
              n130 = call "Build_ERD_Header_String_Array.vi"("ERD Name Array In"=w576, "ERD Number Array In"=w575, "ERD Name List"=string[] ["Drum Light"], "New Header?"=w571, "ERD Number"=w570) -> ("ERD Name Array Out"=w574:string[], "ERD Number Array Out"=w573:string[])  [unwired: 13 in]
              n131 = Insert Into Array(array=w569, new element=w566) -> (w568:string[])  [unwired: 1 in]
              n132 = Bundle By Name(cluster=w579, "Drum Light"=w565) -> (w578:T3)
            }
            frame 61455 {
              n133 = Decimal String To Number(string=w592) -> (number=w591:i32)  [unwired: 2 in, 1 out]
              n134 = Number To Boolean Array(number=w591) -> (Boolean array=w590:bool[])
              n135 = Index Array(array=w590) -> (element #2=w587:bool, element #6=w586:bool, element #8=w584:bool)  [unwired: 8 in, 5 out]
              n136 = case shown="True" w584 {
                tunnel: ["OFF" "ON"] -> w585
                frame False {
                }
                frame True {
                }
              }
              n137 = case shown="True" w587 {
                tunnel: ["OFF" "ON"] -> w589
                frame False {
                }
                frame True {
                }
              }
              n138 = case shown="True" w586 {
                tunnel: ["OFF" "ON"] -> w588
                frame False {
                }
                frame True {
                }
              }
              n139 = call "Build_ERD_Header_String_Array.vi"("ERD Name Array In"=w598, "ERD Number Array In"=w597, "ERD Name List"=string[] ["Water Heater", "V4 - Hot", "Dry Heater"], "New Header?"=w594, "ERD Number"=w593) -> ("ERD Name Array Out"=w596:string[], "ERD Number Array Out"=w595:string[])  [unwired: 13 in]
              n140 = Insert Into Array(array=w601, new element #1=w589, new element #2=w588, new element #3=w585) -> (w600:string[])  [unwired: 1 in]
              n141 = Bundle By Name(cluster=w604, "Water Heater"=w587, "V4 - Hot"=w586, "Dry Heater"=w584) -> (w603:T3)
            }
            frame 61456 {
              n142 = Decimal String To Number(string=w641) -> (number=w640:i32)  [unwired: 2 in, 1 out]
              n143 = Number To Boolean Array(number=w640) -> (Boolean array=w639:bool[])
              n144 = Index Array(array=w639) -> (element #1=w626:bool, element #2=w634:bool, element #3=w625:bool, element #4=w620:bool, element #5=w615:bool, element #6=w617:bool, element #7=w618:bool, element #8=w614:bool)  [unwired: 8 in]
              n145 = Not(x=w626) -> (.not. x?=w630:bool)
              n146 = Compound Arithmetic op=OR(w620, w617, w618) -> (w619:bool)
              n147 = And(x=w626, y=w625) -> (x .and. y?=w627:bool)
              n148 = And(x=w625, y=w630) -> (x .and. y?=w629:bool)
              n149 = Not(x=w625) -> (.not. x?=w632:bool)
              n150 = And(x=w626, y=w632) -> (x .and. y?=w633:bool)
              n151 = case shown="True" w615 {
                selector: w615 -> [w658 w660]
                tunnel: ["OFF" "ON"] -> w616
                tunnel: [w658 w660] -> w611
                frame False {
                }
                frame True {
                }
              }
              n152 = case shown="True" w614 {
                selector: w614 -> [w654 w656]
                tunnel: ["OFF" "ON"] -> w613
                tunnel: [w654 w656] -> w612
                frame False {
                }
                frame True {
                }
              }
              n153 = case shown="True" w629 {
                selector: w629 -> [w670 w672]
                tunnel: ["OFF" "ON"] -> w636
                tunnel: [w670 w672] -> w628
                frame False {
                }
                frame True {
                }
              }
              n154 = case shown="True" w619 {
                selector: w619 -> [w666 w668]
                tunnel: ["OFF" "ON"] -> w635
                tunnel: [w666 w668] -> w623
                frame False {
                }
                frame True {
                }
              }
              n155 = case shown="True" w627 {
                selector: w627 -> [w662 w664]
                tunnel: ["OFF" "ON"] -> w621
                tunnel: [w662 w664] -> w624
                frame False {
                }
                frame True {
                }
              }
              n156 = case shown="True" w633 {
                selector: w633 -> [w678 w680]
                tunnel: ["OFF" "ON"] -> w638
                tunnel: [w678 w680] -> w631
                frame False {
                }
                frame True {
                }
              }
              n157 = case shown="True" w634 {
                selector: w634 -> [w674 w676]
                tunnel: ["OFF" "ON"] -> w637
                tunnel: [w674 w676] -> w622
                frame False {
                }
                frame True {
                }
              }
              n158 = call "Build_ERD_Header_String_Array.vi"("ERD Name Array In"=w647, "ERD Number Array In"=w646, "ERD Name List"=string[] ["V1 - PreWash", "V2 - Main Wash", "V3 - Bleach", "Drain Pump", "V5 - Fabric Softener", "Dry Fan", "V6 - Condenser Valve"], "New Header?"=w643, "ERD Number"=w642) -> ("ERD Name Array Out"=w645:string[], "ERD Number Array Out"=w644:string[])  [unwired: 13 in]
              n159 = Insert Into Array(array=w650, new element #1=w638, new element #2=w637, new element #3=w636, new element #4=w635, new element #5=w621, new element #6=w616, new element #7=w613) -> (w649:string[])  [unwired: 1 in]
              n160 = Bundle By Name(cluster=w653, "V1 - Prewash"=w631, "V2 - Main Wash"=w622, "V3 - Bleach"=w628, "Drain Pump"=w623, "V5 - Fabric Softener"=w624, "Dry Fan"=w611, "Condenser Valve"=w612) -> (w652:T3)
            }
            frame 61458 {
              n161 = Decimal String To Number(string=w698) -> (number=w684:i32)  [unwired: 2 in, 1 out]
              n162 = Divide(x=w684, y=100) -> (x/y=w682:dbl)
              n163 = call "Build_ERD_Header_String_Array.vi"("ERD Name Array In"=w690, "ERD Number Array In"=w689, "ERD Name List"=string[] ["Pressure Hz"], "New Header?"=w686, "ERD Number"=w685) -> ("ERD Name Array Out"=w688:string[], "ERD Number Array Out"=w687:string[])  [unwired: 13 in]
              n164 = Number To Fractional String(number=w682) -> (F-format string=w694:string)  [unwired: 3 in]
              n165 = Insert Into Array(array=w693, new element=w694) -> (w692:string[])  [unwired: 1 in]
              n166 = Bundle By Name(cluster=w697, "Pressure kHZ"=w682) -> (w696:T3)
            }
            frame 61460 {
              w720 = 2 ("length (rest)")
              n167 = String Subset(string=w704, offset (0)=0 ("length (rest)"), length (rest)=w720) -> (substring=w756:string)
              n168 = String Subset(string=w704, offset (0)=3 ("length (rest)"), length (rest)=w720) -> (substring=w752:string)
              n169 = String Subset(string=w704, offset (0)=6 ("length (rest)"), length (rest)=w720) -> (substring=w747:string)
              n170 = String Subset(string=w704, offset (0)=9 ("length (rest)"), length (rest)=w720) -> (substring=w746:string)
              n171 = String Subset(string=w704, offset (0)=12 ("length (rest)"), length (rest)=w720) -> (substring=w729:string)
              n172 = String Subset(string=w704, offset (0)=15 ("length (rest)"), length (rest)=w720) -> (substring=w724:string)
              n173 = String Subset(string=w704, offset (0)=18 ("length (rest)"), length (rest)=w720) -> (substring=w723:string)
              n174 = String Subset(string=w704, offset (0)=21 ("length (rest)")) -> (substring=w708:string)  [unwired: 1 in]
              n175 = String Subset(string=w704, offset (0)=24 ("length (rest)")) -> (substring=w705:string)  [unwired: 1 in]
              n176 = Hexadecimal String To Number(string=w756) -> (number=w751:u32)  [unwired: 2 in, 1 out]
              n177 = Hexadecimal String To Number(string=w752) -> (number=w750:u32)  [unwired: 2 in, 1 out]
              n178 = Hexadecimal String To Number(string=w747) -> (number=w749:u32)  [unwired: 2 in, 1 out]
              n179 = Hexadecimal String To Number(string=w746) -> (number=w748:u32)  [unwired: 2 in, 1 out]
              n180 = Hexadecimal String To Number(string=w729) -> (number=w728:u32)  [unwired: 2 in, 1 out]
              n181 = Hexadecimal String To Number(string=w724) -> (number=w725:u32)  [unwired: 2 in, 1 out]
              n182 = Hexadecimal String To Number(string=w723) -> (number=w722:u32)  [unwired: 2 in, 1 out]
              n183 = Hexadecimal String To Number(string=w708) -> (number=w709:u32)  [unwired: 2 in, 1 out]
              n184 = Hexadecimal String To Number(string=w705) -> (number=w707:u32)  [unwired: 2 in, 1 out]
              n185 = Number To Decimal String(number=w751) -> (decimal integer string=w740:string)  [unwired: 1 in]
              n186 = Number To Decimal String(number=w750) -> (decimal integer string=w739:string)  [unwired: 1 in]
              n187 = Number To Decimal String(number=w749) -> (decimal integer string=w717:string)  [unwired: 1 in]
              n188 = Number To Decimal String(number=w748) -> (decimal integer string=w716:string)  [unwired: 1 in]
              n189 = Number To Decimal String(number=w728) -> (decimal integer string=w715:string)  [unwired: 1 in]
              n190 = Number To Decimal String(number=w725) -> (decimal integer string=w714:string)  [unwired: 1 in]
              n191 = Number To Decimal String(number=w722) -> (decimal integer string=w702:string)  [unwired: 1 in]
              n192 = Number To Decimal String(number=w709) -> (decimal integer string=w701:string)  [unwired: 1 in]
              n193 = Number To Decimal String(number=w707) -> (decimal integer string=w699:string)  [unwired: 1 in]
              n194 = call "Build_ERD_Header_String_Array.vi"("ERD Name Array In"=w735, "ERD Number Array In"=w711, "ERD Name List"=string[] ["UI Verion", "MC Version", "Inv Version", "Personality"], "New Header?"=w732, "ERD Number"=w731) -> ("ERD Name Array Out"=w734:string[], "ERD Number Array Out"=w733:string[])  [unwired: 13 in]
              n195 = Concatenate Strings(w702, "." ("element"), w701) -> (w700:string)
              n196 = Concatenate Strings(w715, "." ("element"), w714) -> (w712:string)
              n197 = Concatenate Strings(w717, "." ("element"), w716) -> (w713:string)
              n198 = Concatenate Strings(w740, "." ("element"), w739) -> (w730:string)
              n199 = Bundle By Name(cluster=w744, "UI - Critical Major"=w740, "UI - Critical Minor"=w739, "UI - Non-Critical Major"=w717, "UI - Non-Critical Minor"=w716, "MC Major"=w715, "MC Minor"=w714, "Inverter Version Major"=w702, "Inverter Version  Minor"=w701, "Model Setting"=w699) -> (w743:T2)
              n200 = Insert Into Array(array=w738, new element #1=w730, new element #2=w713, new element #3=w712, new element #4=w700, new element #5=w699) -> (w737:string[])  [unwired: 1 in]
            }
            frame 61461 {
              n201 = Decimal String To Number(string=w773) -> (number=w759:i32)  [unwired: 2 in, 1 out]
              n202 = Divide(x=w759, y=10) -> (x/y=w757:dbl)
              n203 = call "Build_ERD_Header_String_Array.vi"("ERD Name Array In"=w765, "ERD Number Array In"=w764, "ERD Name List"=string[] ["Inlet Thermistor"], "New Header?"=w761, "ERD Number"=w760) -> ("ERD Name Array Out"=w763:string[], "ERD Number Array Out"=w762:string[])  [unwired: 13 in]
              n204 = Number To Fractional String(number=w757) -> (F-format string=w769:string)  [unwired: 3 in]
              n205 = Insert Into Array(array=w768, new element=w769) -> (w767:string[])  [unwired: 1 in]
              n206 = Bundle By Name(cluster=w772, "Inlet Themistor"=w757) -> (w771:T3)
            }
            frame 61462 {
              n207 = Decimal String To Number(string=w790) -> (number=w776:i32)  [unwired: 2 in, 1 out]
              n208 = Divide(x=w776, y=10) -> (x/y=w774:dbl)
              n209 = call "Build_ERD_Header_String_Array.vi"("ERD Name Array In"=w782, "ERD Number Array In"=w781, "ERD Name List"=string[] ["Outlet Thermistor"], "New Header?"=w778, "ERD Number"=w777) -> ("ERD Name Array Out"=w780:string[], "ERD Number Array Out"=w779:string[])  [unwired: 13 in]
              n210 = Number To Fractional String(number=w774) -> (F-format string=w786:string)  [unwired: 3 in]
              n211 = Insert Into Array(array=w785, new element=w786) -> (w784:string[])  [unwired: 1 in]
              n212 = Bundle By Name(cluster=w789, "Outlet Thermistor"=w774) -> (w788:T3)
            }
            frame Default {
            }
          }
        }
        n213 = in-place-cluster #1("CSV File String Arrays.ERD Name Array"=w14, "CSV File String Arrays.ERD Number Array"=w13, "Version"=w21, "ERD_Always Show"=w20, "CSV File String Arrays.ERD Converted String Data"=w15) -> (w8:T1)
      }
    }
    frame Error {
      n214 = Unbundle By Name(w798) -> ("code"=w802:i32, "status"=w803:bool, "source"=w800:string)
      n215 = Equal?(x=w802, y=-5006) -> (x = y?=w806:bool)
      n216 = case shown="True" w806 {
        tunnel: [w810 FALSE] -> w804
        tunnel: w803 -> [w810 _]
        tunnel: w802 -> [w809 w812]
        tunnel: [w809 w812] -> w801
        tunnel: [w808 w811] -> w799
        tunnel: w800 -> [w808 w811]
        frame False {
        }
        frame True {
        }
      }
      n217 = Bundle By Name(cluster=errorcluster {"status"=FALSE, "code"=0, "source"=""} ("error constant"), "status"=w804, "code"=w801, "source"=w799) -> (w797:errorcluster)
    }
  }
  "Error Out" <- w4
  "All_ERD_Data_Bundled_Brass" <- w3
